vi "IMAQ-RGBtoLuma.vi"(1 "Blue 2D Array":dbl[][](array[numeric]), 2 "Green 2D Array":dbl[][](array[numeric]), 3 "Red 2D Array":dbl[][](array[numeric])) -> (0 "Luma 2D Array":dbl[][](array[numeric]))   [LabVIEW 2010]
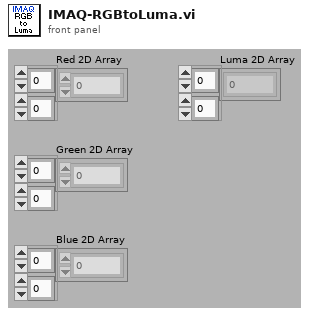
[diagram p1: front panel]
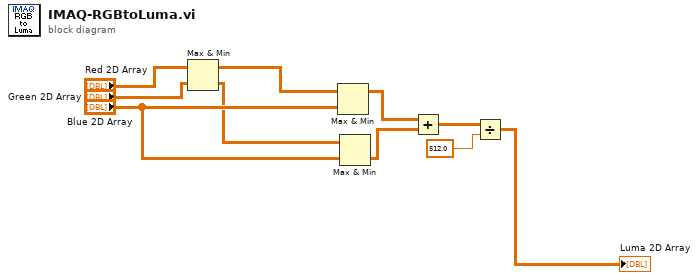
[diagram p0: block diagram]
diagram:
  n1 = Max & Min(x="Red 2D Array", y="Green 2D Array") -> (max(x,y)=w1:dbl[][], min(x,y)=w2:dbl[][])
  n2 = Max & Min(x=w1, y="Blue 2D Array") -> (max(x,y)=w4:dbl[][])  [unwired: 1 out]
  n3 = Max & Min(x=w2, y="Blue 2D Array") -> (min(x,y)=w5:dbl[][])  [unwired: 1 out]
  n4 = Add(x=w4, y=w5) -> (x+y=w6:dbl[][])
  n5 = Divide(x=w6, y=512.0) -> (x/y=→"Luma 2D Array":dbl[][])
